vi "Close.vi"(8 "error in (no error)":errorcluster) -> (0 "error out":errorcluster)   [LabVIEW 2019]
uses:
  <vilib>/Utility/error.llb/Error Cluster From Error Code.vi
  <vilib>/ErrorRing/Error Ring.xnode
  source/repos/Kinova Labview Interface/Debug/KLInterface.dll
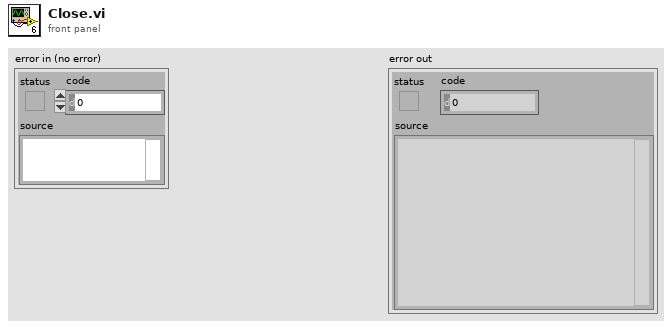
[diagram p1: front panel]
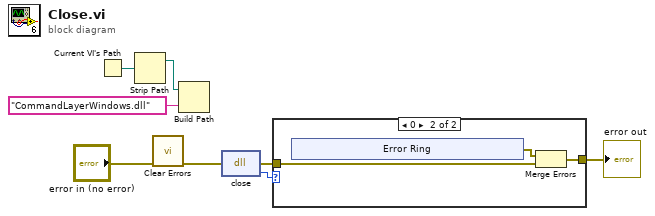
[diagram p0: block diagram]
diagram:
  n1 = Current VI's Path() -> (path=w5:path)
  n2 = Strip Path(path=w5) -> (stripped path=w4:path)  [unwired: 1 out]
  n3 = call <vilib>:"Clear Errors.vi"("error in (no error)"="error in (no error)") -> ("error out"=w1:errorcluster)  [unwired: 5 in, 1 out]
  n4 = Build Path(base path=w4, name or relative path="CommandLayerWindows.dll") -> ()  [unwired: 1 out]
  n5 = dll-call lib="C:/Users/mcjssdcc/source/repos/Kinova Labview Interface/Debug/KLInterface.dll" fn="close"(error in=w1) -> (error out=w7:errorcluster, "return type"=w6:i32)  [unwired: 2 in, 1 out]
  n6 = case shown="0" w6 {
    tunnel: [w9 w11] -> w3
    tunnel: w7 -> [w9 w10]
    frame 1, Default {
    }
    frame 0 {
      n7 = xnode "Error Ring"() -> ("error out"=w12:errorcluster)
      n8 = Merge Errors(w12, w10) -> (w11:errorcluster)
    }
  }
  "error out" <- w3
